vi "TH260_AllDllFunctions_AnyThread.vi"   [LabVIEW 2010]
uses:
  th260lib_x86_x64_AnyThread.llb/TH260_DllPath_global.vi
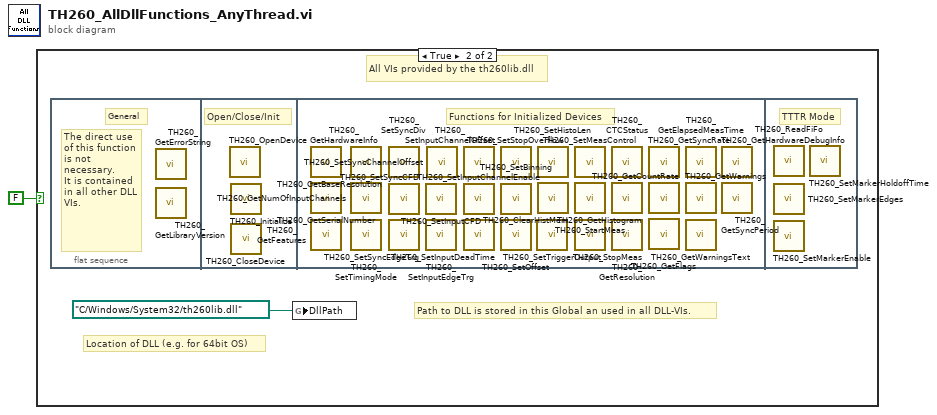
[diagram p0: block diagram]
diagram:
  n1 = case shown="True" FALSE {
    frame False {
    }
    frame True {
      # "Location of DLL (e.g. for 64bit OS)"
      # "Path to DLL is stored in this Global an used in all DLL-VIs."
      # "All VIs provided by the th260lib.dll"
      n2 = flat-sequence {
        frame #0 {
          # "The direct use of this function is not necessary.\nIt is contained in all other DLL VIs."
          # "General"
          n3 = call "TH260_GetErrorString.vi"() -> ()  [unwired: 9 in, 3 out]
          n4 = call "TH260_GetLibraryVersion.vi"() -> ()  [unwired: 9 in, 3 out]
        }
        frame #1 {
          # "Open/Close/Init"
          n5 = call "TH260_OpenDevice.vi"() -> ()  [unwired: 9 in, 3 out]
          n6 = call "TH260_Initialize.vi"() -> ()  [unwired: 10 in, 2 out]
          n7 = call "TH260_CloseDevice.vi"() -> ()  [unwired: 10 in, 2 out]
        }
        frame #2 {
          # "Functions for Initialized Devices"
          n8 = call "TH260_GetHardwareInfo.vi"() -> ()  [unwired: 7 in, 5 out]
          n9 = call "TH260_GetSerialNumber.vi"() -> ()  [unwired: 9 in, 3 out]
          n10 = call "TH260_GetFeatures.vi"() -> ()  [unwired: 9 in, 3 out]
          n11 = call "TH260_GetBaseResolution.vi"() -> ()  [unwired: 8 in, 4 out]
          n12 = call "TH260_GetNumOfInputChannels.vi"() -> ()  [unwired: 9 in, 3 out]
          n13 = call "TH260_SetTimingMode.vi"() -> ()  [unwired: 10 in, 2 out]
          n14 = call "TH260_SetSyncDiv.vi"() -> ()  [unwired: 10 in, 2 out]
          n15 = call "TH260_SetSyncCFD.vi"() -> ()  [unwired: 10 in, 2 out]
          n16 = call "TH260_SetSyncEdgeTrg.vi"() -> ()  [unwired: 10 in, 2 out]
          n17 = call "TH260_SetInputCFD.vi"() -> ()  [unwired: 10 in, 2 out]
          n18 = call "TH260_SetInputEdgeTrg.vi"() -> ()  [unwired: 10 in, 2 out]
          n19 = call "TH260_SetSyncChannelOffset.vi"() -> ()  [unwired: 10 in, 2 out]
          n20 = call "TH260_SetInputChannelOffset.vi"() -> ()  [unwired: 10 in, 2 out]
          n21 = call "TH260_SetInputChannelEnable.vi"() -> ()  [unwired: 10 in, 2 out]
          n22 = call "TH260_SetInputDeadTime.vi"() -> ()  [unwired: 10 in, 2 out]
          n23 = call "TH260_SetStopOverflow.vi"() -> ()  [unwired: 10 in, 2 out]
          n24 = call "TH260_SetBinning.vi"() -> ()  [unwired: 10 in, 2 out]
          n25 = call "TH260_SetOffset.vi"() -> ()  [unwired: 10 in, 2 out]
          n26 = call "TH260_SetTriggerOutput.vi"() -> ()  [unwired: 10 in, 2 out]
          n27 = call "TH260_SetHistoLen.vi"() -> ()  [unwired: 9 in, 3 out]
          n28 = call "TH260_ClearHistMem.vi"() -> ()  [unwired: 10 in, 2 out]
          n29 = call "TH260_SetMeasControl.vi"() -> ()  [unwired: 10 in, 2 out]
          n30 = call "TH260_StartMeas.vi"() -> ()  [unwired: 10 in, 2 out]
          n31 = call "TH260_StopMeas.vi"() -> ()  [unwired: 10 in, 2 out]
          n32 = call "TH260_CTCStatus.vi"() -> ()  [unwired: 9 in, 3 out]
          n33 = call "TH260_GetHistogram.vi"() -> ()  [unwired: 8 in, 3 out]
          n34 = call "TH260_GetResolution.vi"() -> ()  [unwired: 9 in, 3 out]
          n35 = call "TH260_GetSyncRate.vi"() -> ()  [unwired: 9 in, 3 out]
          n36 = call "TH260_GetCountRate.vi"() -> ()  [unwired: 9 in, 3 out]
          n37 = call "TH260_GetFlags.vi"() -> ()  [unwired: 9 in, 3 out]
          n38 = call "TH260_GetElapsedMeasTime.vi"() -> ()  [unwired: 9 in, 3 out]
          n39 = call "TH260_GetWarnings.vi"() -> ()  [unwired: 9 in, 3 out]
          n40 = call "TH260_GetWarningsText.vi"() -> ()  [unwired: 9 in, 3 out]
          n41 = call "TH260_GetHardwareDebugInfo.vi"() -> ()  [unwired: 9 in, 3 out]
          n42 = call "TH260_GetSyncPeriod.vi"() -> ()  [unwired: 9 in, 3 out]
        }
        frame #3 {
          # "TTTR Mode"
          n43 = call "TH260_ReadFiFo.vi"() -> ()  [unwired: 8 in, 4 out]
          n44 = call "TH260_SetMarkerEdges.vi"() -> ()  [unwired: 10 in, 2 out]
          n45 = call "TH260_SetMarkerEnable.vi"() -> ()  [unwired: 10 in, 2 out]
          n46 = call "TH260_SetMarkerHoldoffTime.vi"() -> ()  [unwired: 10 in, 2 out]
        }
      }
      n47 = global write "TH260_DllPath_global.vi" "DllPath"(path "C:/Windows/System32/th260lib.dll" ("DllPath")) -> ()
    }
  }
